vi "RectWHtoRect.vi"() -> (3 "rect":T2 caption="矩形")   [LabVIEW 2011]
uses:
  RectWH/RectWH.ctl
panel:
  in  "RectWH":T1
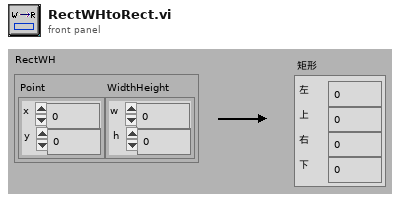
[diagram p1: front panel]
types:
  T1 = typedef "RectWH.ctl" = cluster{"Point":cluster{"x":i16, "y":i16}, "WidthHeight":cluster{"x":i16, "y":i16}}
  T2 = cluster{"left":i16, "top":i16, "right":i16, "bottom":i16}
  T3 = cluster{"Point":cluster{"x":i16, "y":i16}, cluster{"x":i16, "y":i16}}
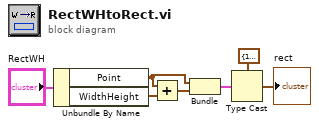
[diagram p0: block diagram]
diagram:
  n1 = Unbundle By Name("RectWH") -> ("Point"=w5:cluster{"x":i16, "y":i16}, "WidthHeight"=w4:cluster{"x":i16, "y":i16})
  n2 = Add(x=w5, y=w4) -> (x+y=w1:cluster{"x":i16, "y":i16})
  n3 = Bundle("Point"=w5, w1) -> (w3:T3)  [unwired: 1 in]
  n4 = Type Cast(type=T2 {"left"=10, "top"=10, "right"=30, "bottom"=50} ("rect"), x=w3) -> (*(type *) &x=→"rect":T2)
